vi "libra_buildup.vi"() -> ()   [LabVIEW 2013]
uses:
  <vilib>/Analysis/baseanly.llb/Mean (DBL).vi
  <vilib>/Analysis/8numeric.llb/1D Numeric Integration.vi
  <vilib>/Analysis/NI_AALPro.lvlib
  <vilib>/Analysis/NI_AALBase.lvlib
panel:
  in  "?":bool
  out "error out":errorcluster
  out "amp":dynamicdata(graph)=[{"t0"=timestamp(3497005917.1967473 s since 1904-01-01), "dt"=1.0, "Y"=[0.0]}, {"t0"=timestamp(3497005917.1967473 s since 1904-01-01), "dt"=1.0, "Y"=[0.0]}]
  out "area":dynamicdata(graph)=[{"t0"=timestamp(3497005917.1967473 s since 1904-01-01), "dt"=1.0, "Y"=[0.15300000000000002]}, {"t0"=timestamp(3497005917.1967473 s since 1904-01-01), "dt"=1.0, "Y"=[0.36000000000000004]}]
  in  "Threshold (%)":dbl=85.0
  out "Area":bool
  out "Area":dbl=0.36000000000000004
  out "Amplitude":bool
  out "Amplitude":dbl
  out "Data":waveform(dbl)(graph)={"t0"=timestamp(-9.000000000813912e-08 s since 1904-01-01), "dt"=4e-11, "Y"=[]}
  in  "Source (0: Channel 1)":u16(ring)=1 items=["Channel 1", "Channel 2", "Channel 3", "Channel 4", "Math", "Reference A", "Reference B", "Reference C", "Reference D", "FFT"]
  in  "Serial Configuration":T1={"Baud Rate"=9600, "Parity"=0, "Stop Bits"=10, "Flow Control"=2} {"Flow Control" items=["None", "XON/XOFF", "RTS/CTS", "XON/XOFF & RTS/CTS", "DTR/DSR", "XON/XOFF & DTR/DSR"]; "Stop Bits" items=["1.0"=10, "1.5"=15, "2.0"=20]; "Parity" items=["None", "Odd", "Even", "Mark", "Space"]; "Baud Rate" items=["300"=300, "600"=600, "1200"=1200, "2400"=2400, "4800"=4800, "9600"=9600, "19200"=19200]}
  in  "VISA resource name":refnum<visa-resource-name>="COM4"
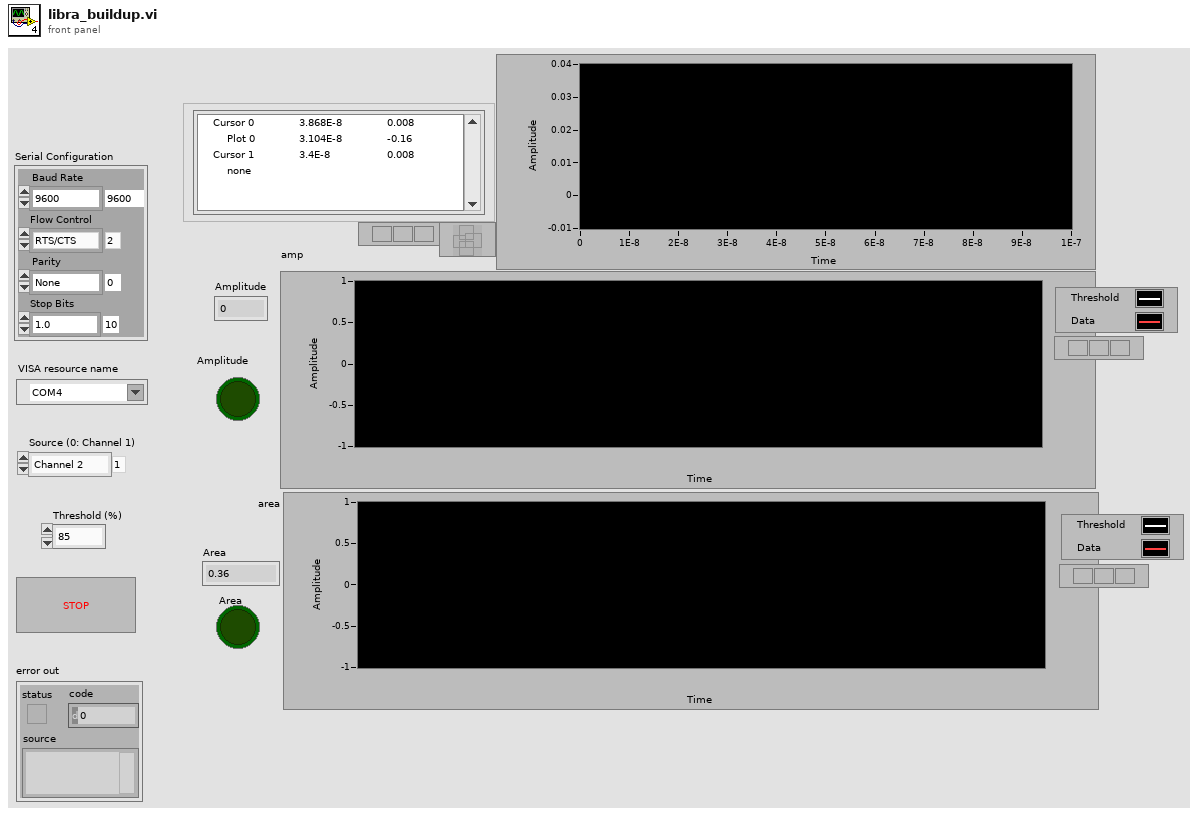
[diagram p1: front panel]
types:
  T1 = cluster{"Baud Rate":u32, "Parity":u16, "Stop Bits":u16, "Flow Control":u16}
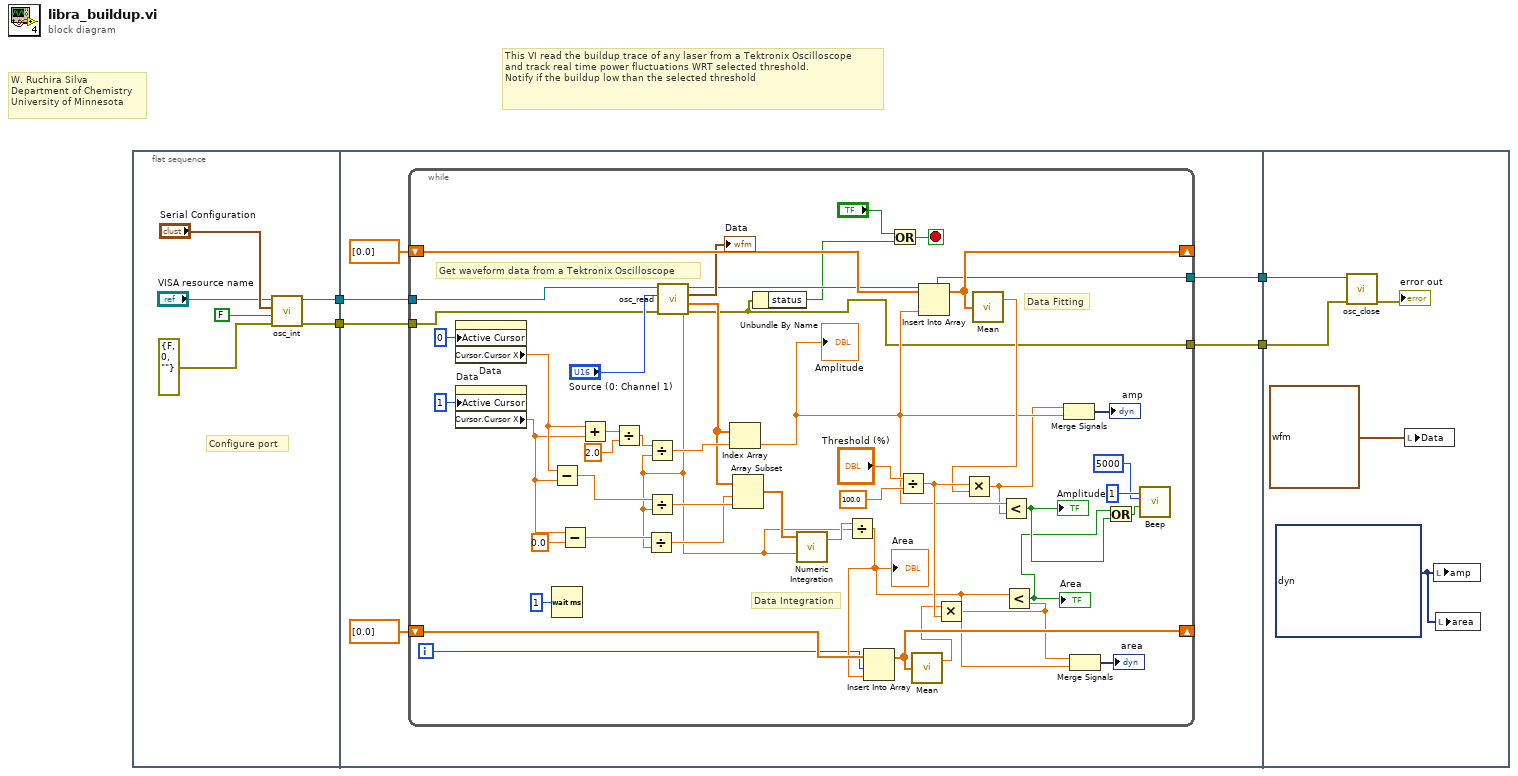
[diagram p0: block diagram]
diagram:
  # "This VI read the buildup trace of any laser from a Tektronix Oscilloscope\nand track real time power fluctuations WRT selected threshold. \nNotify if the buildup low than the selected threshold"
  # "W. Ruchira Silva\nDepartment of Chemistry\nUniversity of Minnesota"
  n1 = flat-sequence {
    tunnel: [w10] -> w4
    tunnel: [w9] -> w3
    tunnel: w4 -> [w16]
    tunnel: w3 -> [w13]
    tunnel: [w12] -> w2
    tunnel: [w11] -> w1
    tunnel: w2 -> [w68]
    tunnel: w1 -> [w67]
    frame #0 {
      # "Configure port"
      n2 = call "osc_int.vi"("VISA resource name"="VISA resource name", "Serial Configuration"="Serial Configuration", "ID Query? (T: Yes)"=FALSE ("Reset? (T: Yes)"), "error in (no error)"=errorcluster {"status"=FALSE, "code"=0, "source"=""}) -> ("VISA resource name out"=w10:refnum<visa-resource-name>, "error out"=w9:errorcluster)  [unwired: 5 in]
    }
    frame #1 {
      n3 = while {
        shift-right: [w33] -> _
        shift-left: dbl[] [0.0] -> [w34]
        shift-right: [w41] -> _
        shift-left: dbl[] [0.0] -> [w42]
        tunnel: w16 -> [w23]
        tunnel: w13 -> [w22]
        tunnel: [w21] -> w12
        tunnel: [w20] -> w11
        i -> [w35]
        stop <- w17 stop-if-true
        # "Data Integration"
        # "Data Fitting"
        # "Get waveform data from a Tektronix Oscilloscope"
        n4 = property on="Data" class="WFGraph (strict)"("Active Cursor"=u32 0) -> ("Cursor.Cursor X"=w58:dbl)  [unwired: 2 in, 2 out]
        n5 = property on="Data" class="WFGraph (strict)"("Active Cursor"=u32 1) -> ("Cursor.Cursor X"=w55:dbl)  [unwired: 2 in, 2 out]
        n6 = Subtract(x=w58, y=w55) -> (x-y=w57:dbl)
        n7 = Wait (ms)(milliseconds to wait=u32 1) -> ()  [unwired: 1 out]
        n8 = Subtract(x=w55, y=0.0) -> (x-y=w54:dbl)
        n9 = Add(x=w58, y=w55) -> (x+y=w62:dbl)
        n10 = Divide(x=w62, y=2.0) -> (x/y=w60:dbl)
        n11 = call "osc_read.vi"("error in (no error)"=w22, "Source (0: Channel 1)"="Source (0: Channel 1)", "VISA resource name"=w23) -> ("error out"=w20:errorcluster, "Y"=w24:dbl[], "Waveform Data"=→"Data":waveform(dbl), "VISA resource name out"=w21:refnum<visa-resource-name>, "dt"=w26:dbl)  [unwired: 3 in, 1 out]
        n12 = Divide(x=w54, y=w26) -> (x/y=w53:dbl)
        n13 = Divide(x=w60, y=w26) -> (x/y=w59:dbl)
        n14 = Divide(x=w57, y=w26) -> (x/y=w56:dbl)
        n15 = Index Array(array=w24, index=w59) -> (element=w29:dbl)
        "Amplitude" <- w29
        n16 = Array Subset(array=w24, index=w53, length=w56) -> (w52:dbl[])
        n17 = Unbundle By Name(w20) -> ("status"=w19:bool)
        n18 = call-poly <vilib>:"Numeric Integration.vi"("dt"=w26, "Input Array"=w52) -> ("result"=w43:dbl)  [unwired: 1 in, 1 out]
        n19 = Divide(x=w43, y=w26) -> (x/y=w36:dbl)
        "Area" <- w36
        n20 = Insert Into Array(array=w42, index=w35, new element=w36) -> (w41:dbl[])
        n21 = Or(x="?", y=w19) -> (x .or. y?=w17:bool)
        n22 = Divide(x="Threshold (%)", y=100.0) -> (x/y=w44:dbl)
        n23 = call-poly <vilib>:"Mean.vi"("X"=w41) -> ("mean"=w40:dbl)  [unwired: 1 out]
        n24 = Insert Into Array(array=w34, new element=w29) -> (w33:dbl[])  [unwired: 1 in]
        n25 = Multiply(x=w40, y=w44) -> (x*y=w30:dbl)
        n26 = call-poly <vilib>:"Mean.vi"("X"=w33) -> ("mean"=w31:dbl)  [unwired: 1 out]
        n27 = Multiply(x=w44, y=w31) -> (x*y=w28:dbl)
        n28 = Less?(x=w29, y=w28) -> (x < y?=w48:bool)
        "Amplitude" <- w48
        n29 = Less?(x=w36, y=w30) -> (x < y?=w39:bool)
        "Area" <- w39
        n30 = Merge Signals(w28, w29) -> (→"amp":dynamicdata)
        n31 = Merge Signals(w30, w36) -> (→"area":dynamicdata)
        n32 = Or(x=w39, y=w48) -> (x .or. y?=w47:bool)
        n33 = call <vilib>:"Beep.vi"("use system alert? (T)"=w47, "duration (msec)"=u32 5000, "frequency (Hz)"=u32 1) -> ()  [unwired: 9 in]
      }
    }
    frame #2 {
      w66 = dynamicdata [{"t0"=timestamp(3497005917.1967473 s since 1904-01-01), "dt"=1.0, "Y"=[0.0]}, {"t0"=timestamp(3497005917.1967473 s since 1904-01-01), "dt"=1.0, "Y"=[0.0]}] ("amp")
      n34 = call "osc_close.vi"("error in (no error)"=w67, "VISA resource name"=w68) -> ("error out"=→"error out":errorcluster)  [unwired: 9 in]
      n35 = local write "Data"(waveform(dbl) {"t0"=timestamp(-9.000000000813912e-08 s since 1904-01-01), "dt"=4e-11, "Y"=array[2500 elements]} ("Waveform Data")) -> ()
      n36 = local write "amp"(w66) -> ()
      n37 = local write "area"(w66) -> ()
    }
  }
